vi "Vpp to Dbm Acquisition.vi"(10 "address":i16, 11 "bus":i32) -> (3 "Dbm":dbl)   [LabVIEW 2024]
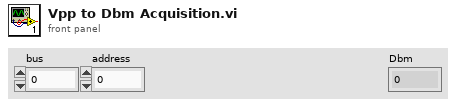
[diagram p1: front panel]
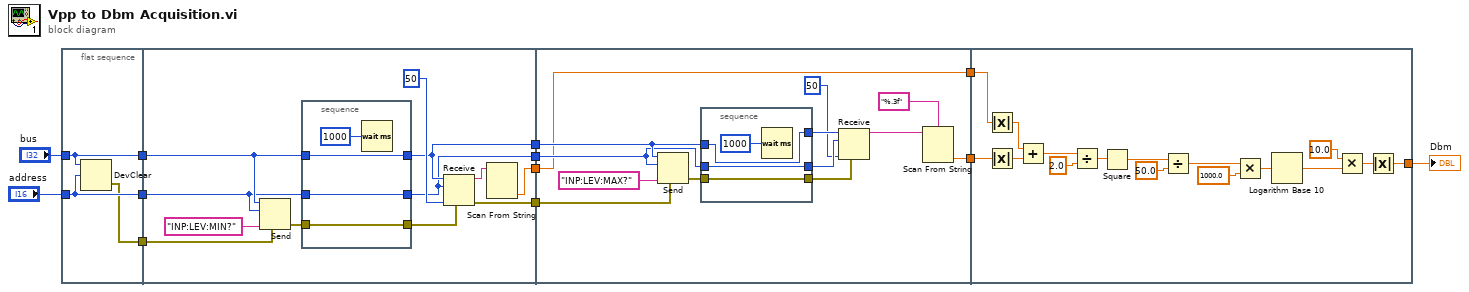
[diagram p0: block diagram]
diagram:
  n1 = flat-sequence {
    tunnel: "address" -> [w14]
    tunnel: "bus" -> [w15]
    tunnel: [w15] -> w3
    tunnel: [w14] -> w2
    tunnel: [w13] -> w1
    tunnel: [w23] -> w12
    tunnel: [w22] -> w9
    tunnel: [w21] -> w8
    tunnel: [w17] -> w4
    tunnel: w3 -> [w20]
    tunnel: w2 -> [w19]
    tunnel: w1 -> [w16]
    tunnel: w12 -> [w37]
    tunnel: [w35] -> w11
    tunnel: w9 -> [w34]
    tunnel: w8 -> [w33]
    tunnel: [w32] -> w5
    tunnel: w4 -> [w32]
    tunnel: w11 -> [w54]
    tunnel: [w49] -> w10
    tunnel: w5 -> [w51]
    frame #0 {
      n2 = DevClear(3:w14, 4:w15) -> (0:w13:errorcluster)  [unwired: 1 in, 1 out]
    }
    frame #1 {
      n3 = Send(0:w20, 2:w19, 4:w16, 5:"INP:LEV:MIN?" ("data string")) -> (8:w26:errorcluster)  [unwired: 1 in, 2 out]
      n4 = stacked-sequence {
        tunnel: w26 -> [w29]
        tunnel: [w30] -> w22
        tunnel: [w31] -> w21
        tunnel: w19 -> [w31]
        tunnel: w20 -> [w30]
        tunnel: [w29] -> w18
        frame #0 {
          n5 = Wait (ms)(milliseconds to wait=u32 1000) -> ()  [unwired: 1 out]
        }
      }
      n6 = Receive(4:w18, 6:50 ("count"), 8:w21, 9:w22) -> (0:w23:errorcluster, 3:w27:string)  [unwired: 1 in, 2 out]
      n7 = Scan From String(input string=w27) -> (output 1=w17:dbl)  [unwired: 4 in, 3 out]
    }
    frame #2 {
      n8 = Send(0:w34, 2:w33, 4:w37, 5:"INP:LEV:MAX?" ("data string")) -> (8:w40:errorcluster)  [unwired: 1 in, 2 out]
      n9 = stacked-sequence {
        tunnel: w40 -> [w46]
        tunnel: [w47] -> w41
        tunnel: [w48] -> w42
        tunnel: w33 -> [w48]
        tunnel: w34 -> [w47]
        tunnel: [w46] -> w43
        frame #0 {
          n10 = Wait (ms)(milliseconds to wait=u32 1000) -> ()  [unwired: 1 out]
        }
      }
      n11 = Receive(4:w43, 6:50 ("count"), 8:w42, 9:w41) -> (3:w44:string)  [unwired: 1 in, 3 out]
      n12 = Scan From String(format string="%.3f" ("Format String"), input string=w44) -> (output 1=w35:dbl)  [unwired: 3 in, 3 out]
    }
    frame #3 {
      n13 = Absolute Value(x=w51) -> (abs(x)=w59:dbl)
      n14 = Absolute Value(x=w54) -> (abs(x)=w60:dbl)
      n15 = Add(x=w59, y=w60) -> (x+y=w61:dbl)
      n16 = Divide(x=w61, y=2.0) -> (x/y=w58:dbl)
      n17 = Square(x=w58) -> (x^2=w62:dbl)
      n18 = Divide(x=w62, y=50.0) -> (x/y=w63:dbl)
      n19 = Multiply(x=w63, y=1000.0) -> (x*y=w64:dbl)
      n20 = Logarithm Base 10(1:w64) -> (0:w53:dbl)
      n21 = Multiply(x=10.0, y=w53) -> (x*y=w50:dbl)
      n22 = Absolute Value(x=w50) -> (abs(x)=w49:dbl)
    }
  }
  "Dbm" <- w10
